vi "Magic Tote Detect.vi"(10 "Image Dst Out":T1) -> ()   [LabVIEW 2014]
uses:
  <vilib>/vision/Image Controls.llb/IMAQ Image.ctl
  <vilib>/vision/NI_Vision_Development_Module.lvlib
panel:
  in  "Zone Size":dbl=7.0 format="%#_13g"
  in  "Exam Zone Offset X":dbl
  in  "Exam Zone Offset Y":dbl
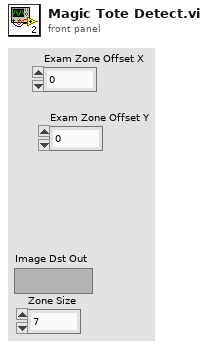
[diagram p1: front panel]
types:
  T1 = typedef "IMAQ Image.ctl" = refnum<image>
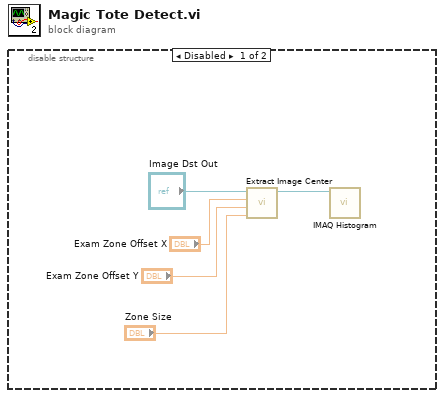
[diagram p0: block diagram]
diagram:
  n1 = disable-structure shown="Disabled" {
    frame Disabled {
      n2 = call "Extract Image Center.vi"("Zone Size"="Zone Size", "Exam Zone Offset Y"="Exam Zone Offset Y", "Exam Zone Offset X"="Exam Zone Offset X", "Source In"="Image Dst Out") -> ("Annotated Source Out"=w1:T1)  [unwired: 6 in, 1 out]
      n3 = call "IMAQ Histogram"("Image"=w1) -> ()  [unwired: 9 in, 2 out]
    }
    frame Enabled {
    }
  }
